vi "LV SciSDK DIGITIZER.vi"(7 "Digitizer Handle In":T3, 9 "Board Handle In":T1, 11 "error in (no error)":errorcluster) -> (4 "NI Error Code":i32, 6 "Digitizer Buffer Out":T2, 8 "Digitizer Handle Out":T3, 10 "Board Handle Out":T1, 15 "error out":errorcluster)   [LabVIEW 2021, in "SciSDK_Labview.lvlib"]
uses:
  SciSDK_Labview.lvlib
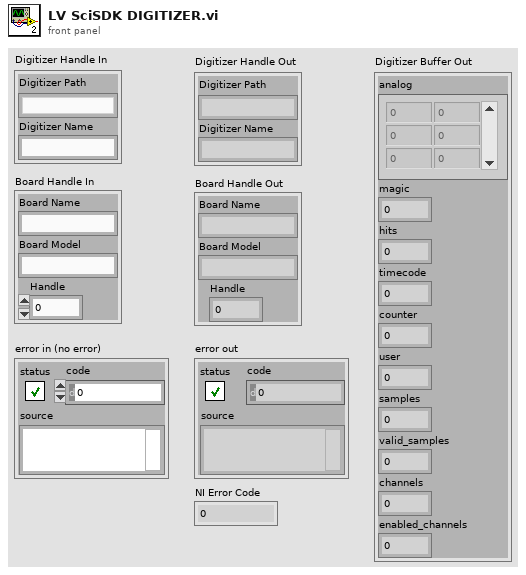
[diagram p1: front panel]
types:
  T1 = cluster{"Board Name":string, "Board Model":string, "Handle":u64}
  T2 = cluster{"analog":i32[][], "magic":u32, "hits":u32, "timecode":u32, "counter":u32, "user":u32, "samples":u32, "valid_samples":u32, "channels":u32, "enabled_channels":u32}
  T3 = cluster{"Digitizer Path":string, "Digitizer Name":string}
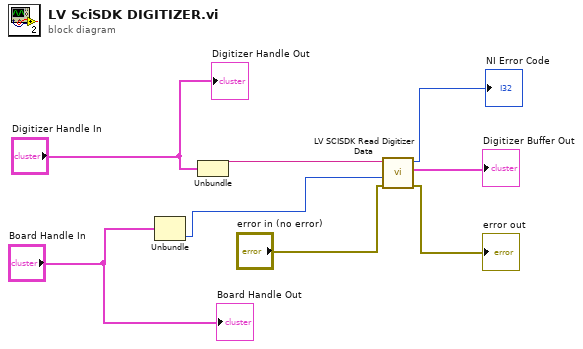
[diagram p0: block diagram]
diagram:
  n1 = Unbundle("Board Handle In") -> ("Handle"=w2:u64)  [unwired: 2 out]
  n2 = Unbundle("Digitizer Handle In") -> ("Digitizer Path"=w3:string)  [unwired: 1 out]
  n3 = call "LV SCISDK Read Digitizer Data.vi"("error in (no error)"="error in (no error)", "handle"=w2, "Path"=w3) -> ("error out"=→"error out":errorcluster, "buffer out"=→"Digitizer Buffer Out":T2, "function return"=→"NI Error Code":i32)  [unwired: 5 in, 1 out]
  "Digitizer Handle Out" <- "Digitizer Handle In"
  "Board Handle Out" <- "Board Handle In"
